vi "Measure and Update Array.vi"(0 "Array In":dbl[][](array[numeric]), 1 "number of samples per channel":i32=-1, 5 "task/channels in":refnum<k21>, 7 "Row":i32, 9 "Column":i32, 11 "error in":errorcluster, 12 "Invert?":bool, 13 "Offset":dbl, 14 "Total Steps in Fast":i32) -> (4 "Array Out":dbl[][](array[numeric]), 6 "task out":refnum<k21>, 8 "Measurement":dbl, 15 "error out":errorcluster)   [LabVIEW 2021]
uses:
  <vilib>/DAQmx/read.llb/DAQmx Read (Analog 1D DBL 1Chan NSamp).vi
  <vilib>/Analysis/baseanly.llb/Mean (DBL).vi
  <vilib>/DAQmx/miscellaneous.llb/DAQmx Fill In Error Info.vi
  <vilib>/Analysis/NI_AALBase.lvlib
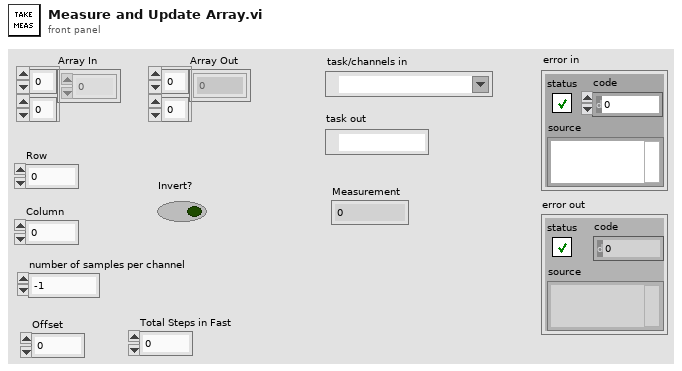
[diagram p1: front panel]
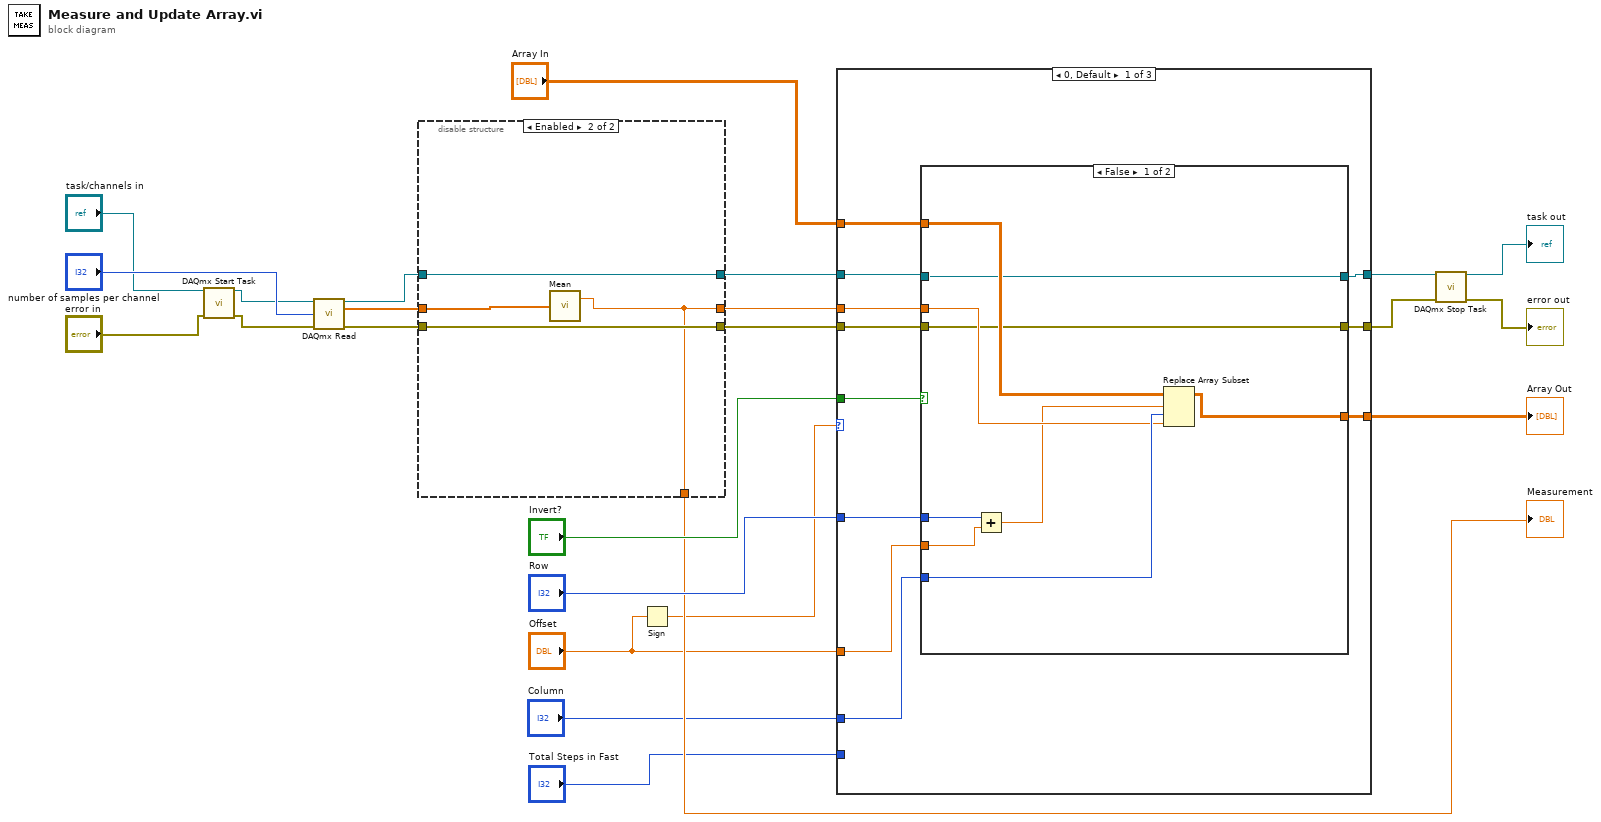
[diagram p0: block diagram]
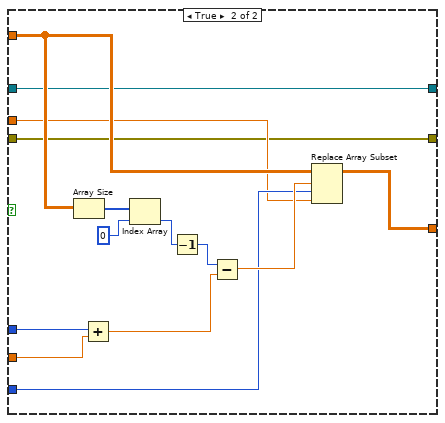
[diagram p2: hidden frame]
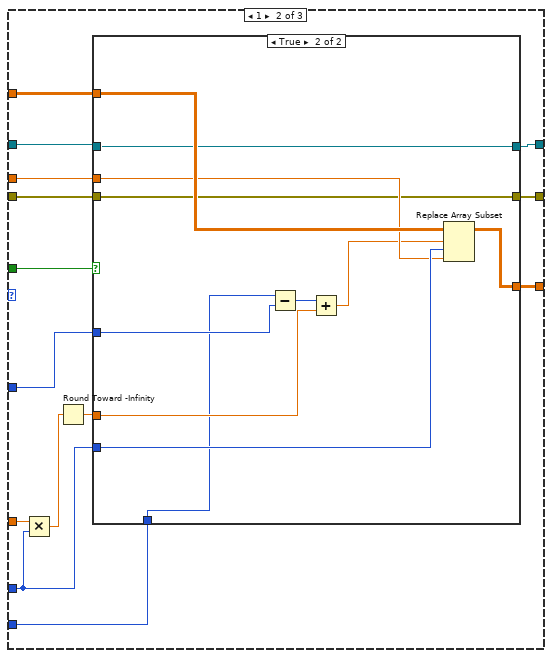
[diagram p3: hidden frame]
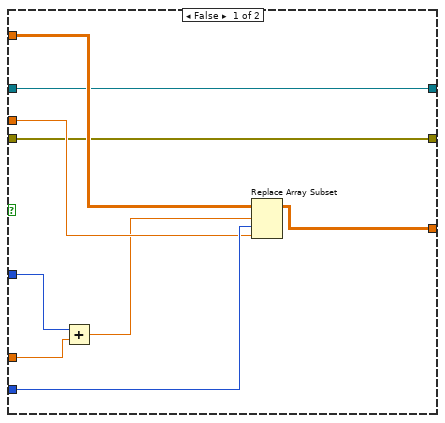
[diagram p4: hidden frame]
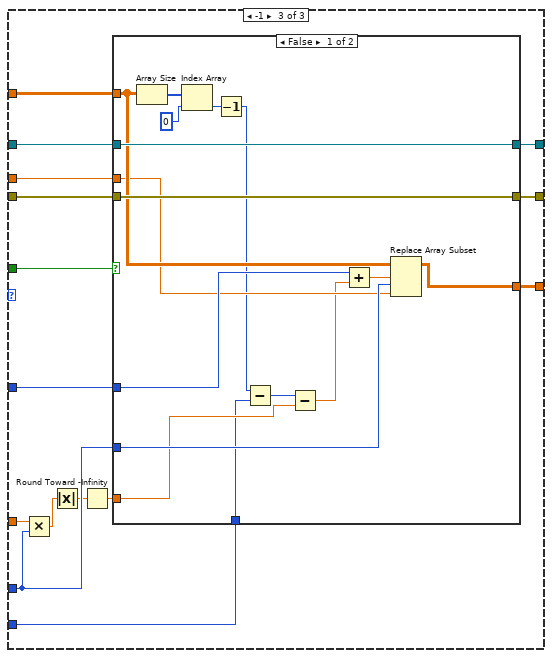
[diagram p5: hidden frame]
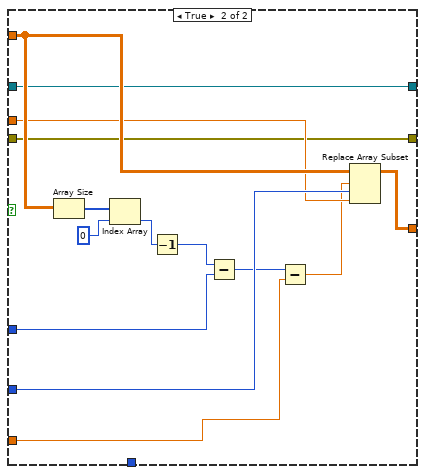
[diagram p6: hidden frame]
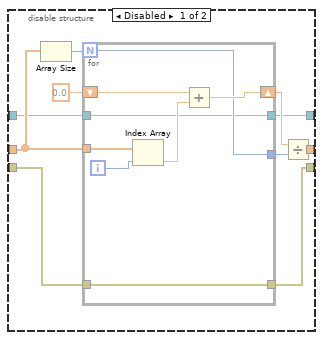
[diagram p7: hidden frame]
diagram:
  n1 = call <vilib>:"DAQmx Start Task.vi"("task/channels in"="task/channels in", "error in"="error in") -> ("task out"=w6:refnum<k21>, "error out"=w9:errorcluster)  [unwired: 12 in]
  n2 = call-poly <vilib>:"DAQmx Read.vi"("task/channels in"=w6, "number of samples per channel"="number of samples per channel", "error in"=w9) -> ("task out"=w10:refnum<k21>, "data"=w17:dbl[], "error out"=w13:errorcluster)  [unwired: 10 in]
  n3 = disable-structure shown="Enabled" {
    disable-tunnel: w17 -> [w33 w46]
    disable-tunnel: [w29 w43] -> w16
    disable-tunnel: [w28 w45] -> w15
    disable-tunnel: [w27 w44] -> w14
    disable-tunnel: w13 -> [w26 w45]
    disable-tunnel: w10 -> [w25 w44]
    disable-tunnel: [_ w43] -> w5
    frame Disabled {
      n4 = Array Size(array=w33) -> (size(s)=w34:i32)
      n5 = for {
        N: w34 -> [w38]
        tunnel: w33 -> [w35]
        shift-right: [w41] -> w30
        shift-left: 0.0 ("Waveform") -> [w39]
        tunnel: [w38] -> w31
        tunnel: w26 -> [w37]
        tunnel: [w37] -> w28
        tunnel: w25 -> [w36]
        tunnel: [w36] -> w27
        i -> [w42]
        n6 = Index Array(array=w35, index=w42) -> (element=w40:dbl)
        n7 = Add(x=w39, y=w40) -> (x+y=w41:dbl)
      }
      n8 = Divide(x=w30, y=w31) -> (x/y=w29:dbl)
    }
    frame Enabled {
      n9 = call-poly <vilib>:"Mean.vi"("X"=w46) -> ("mean"=w43:dbl)  [unwired: 1 out]
    }
  }
  "Measurement" <- w5
  n10 = Sign(1:"Offset") -> (0:w3:dbl)
  n11 = case shown="0, Default" w3 {
    tunnel: "Invert?" -> [w57 w94 w129]
    tunnel: "Array In" -> [w56 w93 w128]
    tunnel: "Column" -> [w55 w84 w119]
    tunnel: "Row" -> [w54 w92 w127]
    tunnel: [w53 w91 w126] -> w21
    tunnel: [w52 w90 w125] -> w20
    tunnel: [w51 w89 w124] -> w19
    tunnel: w16 -> [w50 w88 w123]
    tunnel: w15 -> [w49 w87 w122]
    tunnel: w14 -> [w48 w86 w121]
    tunnel: "Offset" -> [w47 w85 w120]
    tunnel: "Total Steps in Fast" -> [_ w81 w118]
    frame 0, Default {
      n12 = case shown="False" w57 {
        tunnel: w56 -> [w66 w80]
        tunnel: w55 -> [w65 w74]
        tunnel: w54 -> [w60 w69]
        tunnel: [w64 w73] -> w53
        tunnel: w50 -> [w63 w72]
        tunnel: w48 -> [w62 w71]
        tunnel: [w62 w71] -> w52
        tunnel: w49 -> [w61 w70]
        tunnel: [w61 w70] -> w51
        tunnel: w47 -> [w59 w67]
        frame False {
          n13 = Add(x=w60, y=w59) -> (x+y=w58:dbl)
          n14 = Replace Array Subset(array=w66, new element=w63, index (row)=w58, index (col)=w65) -> (w64:dbl[][])
        }
        frame True {
          n15 = Array Size(array=w80) -> (size(s)=w79:i32[])
          n16 = Add(x=w69, y=w67) -> (x+y=w68:dbl)
          n17 = Index Array(array=w79, index=0) -> (element=w77:i32)
          n18 = Decrement(x=w77) -> (x-1=w76:i32)
          n19 = Subtract(x=w76, y=w68) -> (x-y=w75:dbl)
          n20 = Replace Array Subset(array=w80, new element=w72, index (row)=w75, index (col)=w74) -> (w73:dbl[][])
        }
      }
    }
    frame 1 {
      n21 = Multiply(x=w85, y=w84) -> (x*y=w82:dbl)
      n22 = Round Toward -Infinity(1:w82) -> (0:w83:dbl)
      n23 = case shown="True" w94 {
        tunnel: w93 -> [w103 w114]
        tunnel: w84 -> [w102 w113]
        tunnel: w92 -> [w97 w107]
        tunnel: [w101 w112] -> w91
        tunnel: w88 -> [w100 w111]
        tunnel: w86 -> [w99 w110]
        tunnel: [w99 w110] -> w90
        tunnel: w87 -> [w98 w109]
        tunnel: [w98 w109] -> w89
        tunnel: w83 -> [w96 w108]
        tunnel: w81 -> [_ w104]
        frame False {
          n24 = Add(x=w97, y=w96) -> (x+y=w95:dbl)
          n25 = Replace Array Subset(array=w103, new element=w100, index (row)=w95, index (col)=w102) -> (w101:dbl[][])
        }
        frame True {
          n26 = Subtract(x=w104, y=w107) -> (x-y=w106:i32)
          n27 = Add(x=w106, y=w108) -> (x+y=w105:dbl)
          n28 = Replace Array Subset(array=w114, new element=w111, index (row)=w105, index (col)=w113) -> (w112:dbl[][])
        }
      }
    }
    frame -1 {
      n29 = Multiply(x=w120, y=w119) -> (x*y=w116:dbl)
      n30 = Absolute Value(x=w116) -> (abs(x)=w115:dbl)
      n31 = Round Toward -Infinity(1:w115) -> (0:w117:dbl)
      n32 = case shown="False" w129 {
        tunnel: w128 -> [w139 w159]
        tunnel: w119 -> [w145 w156]
        tunnel: w127 -> [w136 w149]
        tunnel: [w144 w155] -> w126
        tunnel: w123 -> [w133 w154]
        tunnel: w121 -> [w143 w153]
        tunnel: [w143 w153] -> w125
        tunnel: w122 -> [w142 w152]
        tunnel: [w142 w152] -> w124
        tunnel: w117 -> [w137 w147]
        tunnel: w118 -> [w134 _]
        frame False {
          n33 = Array Size(array=w139) -> (size(s)=w141:i32[])
          n34 = Index Array(array=w141, index=0) -> (element=w132:i32)
          n35 = Decrement(x=w132) -> (x-1=w131:i32)
          n36 = Subtract(x=w131, y=w134) -> (x-y=w138:i32)
          n37 = Subtract(x=w138, y=w137) -> (x-y=w130:dbl)
          n38 = Add(x=w136, y=w130) -> (x+y=w135:dbl)
          n39 = Replace Array Subset(array=w139, new element=w133, index (row)=w135, index (col)=w145) -> (w144:dbl[][])
        }
        frame True {
          n40 = Array Size(array=w159) -> (size(s)=w158:i32[])
          n41 = Index Array(array=w158, index=0) -> (element=w151:i32)
          n42 = Decrement(x=w151) -> (x-1=w150:i32)
          n43 = Subtract(x=w150, y=w149) -> (x-y=w148:i32)
          n44 = Subtract(x=w148, y=w147) -> (x-y=w146:dbl)
          n45 = Replace Array Subset(array=w159, new element=w154, index (row)=w146, index (col)=w156) -> (w155:dbl[][])
        }
      }
    }
  }
  "Array Out" <- w21
  n46 = call <vilib>:"DAQmx Stop Task.vi"("task/channels in"=w20, "error in"=w19) -> ("task out"=→"task out":refnum<k21>, "error out"=→"error out":errorcluster)  [unwired: 12 in]
